vi "EmgSignalSubVI.vi"(6 "Highpass Cutoff":dbl, 9 "sampling freq: fs":dbl, 10 "Array in":dbl[][](array[numeric]), 11 "filter type":T1) -> (3 "Array out":dbl[][](array[numeric]))   [LabVIEW 2021]
uses:
  <vilib>/Analysis/3filter.llb/Filter Passband Type.ctl
  <vilib>/Analysis/3filter.llb/Butterworth Filter (DBL).vi
  <vilib>/Analysis/NI_AALBase.lvlib
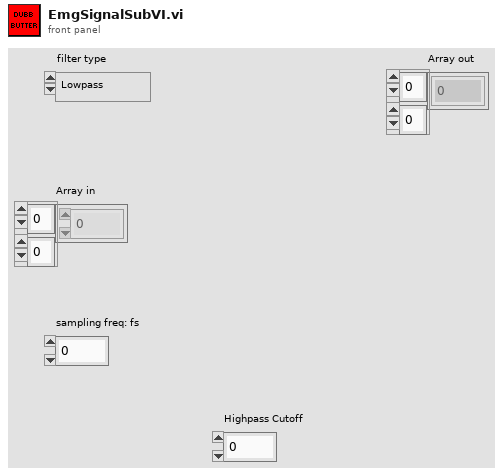
[diagram p1: front panel]
types:
  T1 = typedef "NI_AALBase.lvlib/Filter Passband Type.ctl" = enum32{"Lowpass", "Highpass", "Bandpass", "Bandstop"}
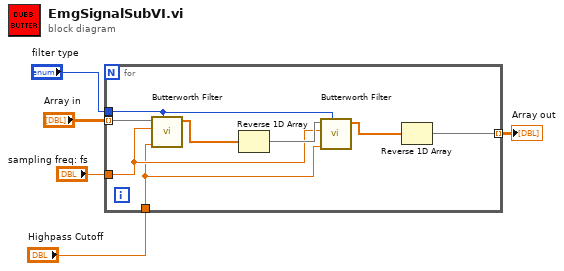
[diagram p0: block diagram]
diagram:
  n1 = for {
    tunnel: "Array in" -> [w10] mode=indexing
    tunnel: "sampling freq: fs" -> [w9]
    tunnel: "Highpass Cutoff" -> [w8]
    tunnel: [w7] -> w4 mode=indexing
    tunnel: "filter type" -> [w6]
    n2 = call-poly <vilib>:"Butterworth Filter.vi"("filter type"=w6, "low cutoff freq: fl"=w8, "sampling freq: fs"=w9, "X"=w10) -> ("Filtered X"=w13:dbl[])  [unwired: 4 in, 1 out]
    n3 = Reverse 1D Array(array=w13) -> (reversed array=w12:dbl[])
    n4 = call-poly <vilib>:"Butterworth Filter.vi"("filter type"=w6, "low cutoff freq: fl"=w8, "sampling freq: fs"=w9, "X"=w12) -> ("Filtered X"=w11:dbl[])  [unwired: 4 in, 1 out]
    n5 = Reverse 1D Array(array=w11) -> (reversed array=w7:dbl[])
  }
  "Array out" <- w4
